vi "Accelerator_DAQ_small.vi"() -> ()   [LabVIEW 2013]
doc: "Acquire Accelerator Data"
uses:
  <instrlib>/niScope/Controls/niScope vertical coupling.ctl
  <instrlib>/niScope/Controls/niScope trigger slope.ctl
  <instrlib>/niScope/Controls/niScope trigger coupling.ctl
  <instrlib>/niScope/Controls/niScope trigger source.ctl
  Accelerator Measurement/Array_Defctl.ctl
  <vilib>/Utility/error.llb/DialogType.ctl
  <vilib>/Utility/miscctls.llb/LVPointTypeDef.ctl
  Public API/Dust_Event.ctl
  Public API/Signal.ctl
  Private/Role ID.ctl
  Private/Hardware ID.ctl
  Private/Estimate_source.ctl
  Functional Global Variables/Action Items.ctl
  <vilib>/Analysis/baseanly.llb/Mean (DBL).vi
  Private/PSU updated.vi
  <vilib>/addons/database/Connection.llb/Conn Execute.vi
  <vilib>/addons/database/Recordset.llb/Rec Fetch Recordset Data (R).vi
  <vilib>/addons/database/Recordset.llb/Rec Destroy - Connection.vi
  <instrlib>/niScope/Configure/Trigger/niScope Configure Trigger Edge.vi
  <instrlib>/niScope/Acquire/Fetch/niScope Multi Fetch Cluster.vi
  <vilib>/addons/database/_DB Variant To Data/Database Variant To Data.xnode
  <vilib>/Analysis/NI_AALBase.lvlib
  <vilib>/addons/database/NI_Database_API.lvlib
panel:
  out "Big Accelerator?":bool
  in  "Trigger":enum32{"Edge"}(tab)
  in  "Trigger Source Edge 2":T1="2" caption="Source"
  in  "Trigger Source Edge":T1="0" caption="Source"
  in  "Coupling":T2=1 items=["AC"=0, "DC"=1, "HF Reject"=3, "LF Reject"=4, "AC Plus HF Reject"=1001]
  in  "Slope":T3 caption="Trigger Slope"
  in  "Level":dbl=1.0 caption="Trigger Level" step=0.001 format="%.3f"
  in  "Delay":dbl caption="Trigger Delay" format="%.4p"
  in  "Reference Position (%)":dbl=40.0 caption="Ref Position" format="%.1f"
  in  "Bandwidth":dbl=-1.0 format="%.2f"
  in  "Vertical Coupling":T4=1 items=["AC", "DC", "Ground"]
  in  "Probe Attenuation":dbl=1.0 format="%.1f"
  in  "Vertical Offset":dbl format="%.4f"
  in  "Vertical Range":dbl=5.0 caption="Vertical Range (V)" format="%.2f"
  out "Actual Sample Rate":dbl=10000000.0 format="%.0p"
  in  "Min Record Length":i32=100000 caption="Min. Record Length"
  in  "Min Sample Rate":dbl=80000000.0 caption="Min. Sample Rate" step=1000000.0 format="%.2p"
  out "Actual Record Length":i32=100000
  out "Mass":dbl format="%#_3g"
  in  "Write to Database?":bool=TRUE
  in  "Limit":dbl
  in  "Limit Triggers":bool
  out "Acquisition #":i32
  in  "WFM Tag":string="trace"
  in  "Location":string="G:\\default"
  in  "Write Raw File?":bool
  out "Saving Raw File...":path=path "G:/2012_06_13_verify_timestamp_labview/trace00000"
  out "?":cluster{dbl, dbl}(knob)={0.0549, 2.0} scale=10.0..0.01
  in  "Ideal Time (Cursor)":dbl=2.0 step=0.01 format="%_2f"
  out "Time Between Triggers":dbl
  out "Average Frequency":dbl format="%#_4g"
  out "output cluster":T5
  out "error out 4":errorcluster
  out "error out 3":errorcluster
  out "# elements in queue":i32
  out "Stop condition":bool=TRUE
  out "created path":path=path "G:/default"
  out "Numeric":i32=92364
  out "error out 2":errorcluster
  out "Calibration":dbl=24700000000000.0
  out "Array":T6=["Dev1", "Dev2"]
  out "Multi Plot 2":cluster{dbl[], dbl[]}(graph) caption="Multi Plot"
  in  "Acceleration Voltage (MV)":dbl=2.0 format="%_2g"
  out "Charge":dbl format="%#_3g"
  out "Velocity (Est.)":dbl format="%#_6f"
  out "Final Detector (CH3)":waveform(dbl)(graph)={"t0"=timestamp(0 s since 1904-01-01), "dt"=1e-07, "Y"=[]}
  out "Charge Detector/PSU gate (CH2)":waveform(dbl)(graph)={"t0"=timestamp(0 s since 1904-01-01), "dt"=1e-07, "Y"=[]}
  out "Velocity Detectors (CH0 & CH1)":waveform(dbl)[](graph)
  in  "stop":bool=TRUE
  out "error out":errorcluster={"status"=FALSE, "code"=0, "source"="No Error"} {"code" format="%.0x"}
  # "File Parameters"
  # "Error Handling"
  # "Trigger"
  # "Channel"
  # "Vertical"
  # "Horizontal"
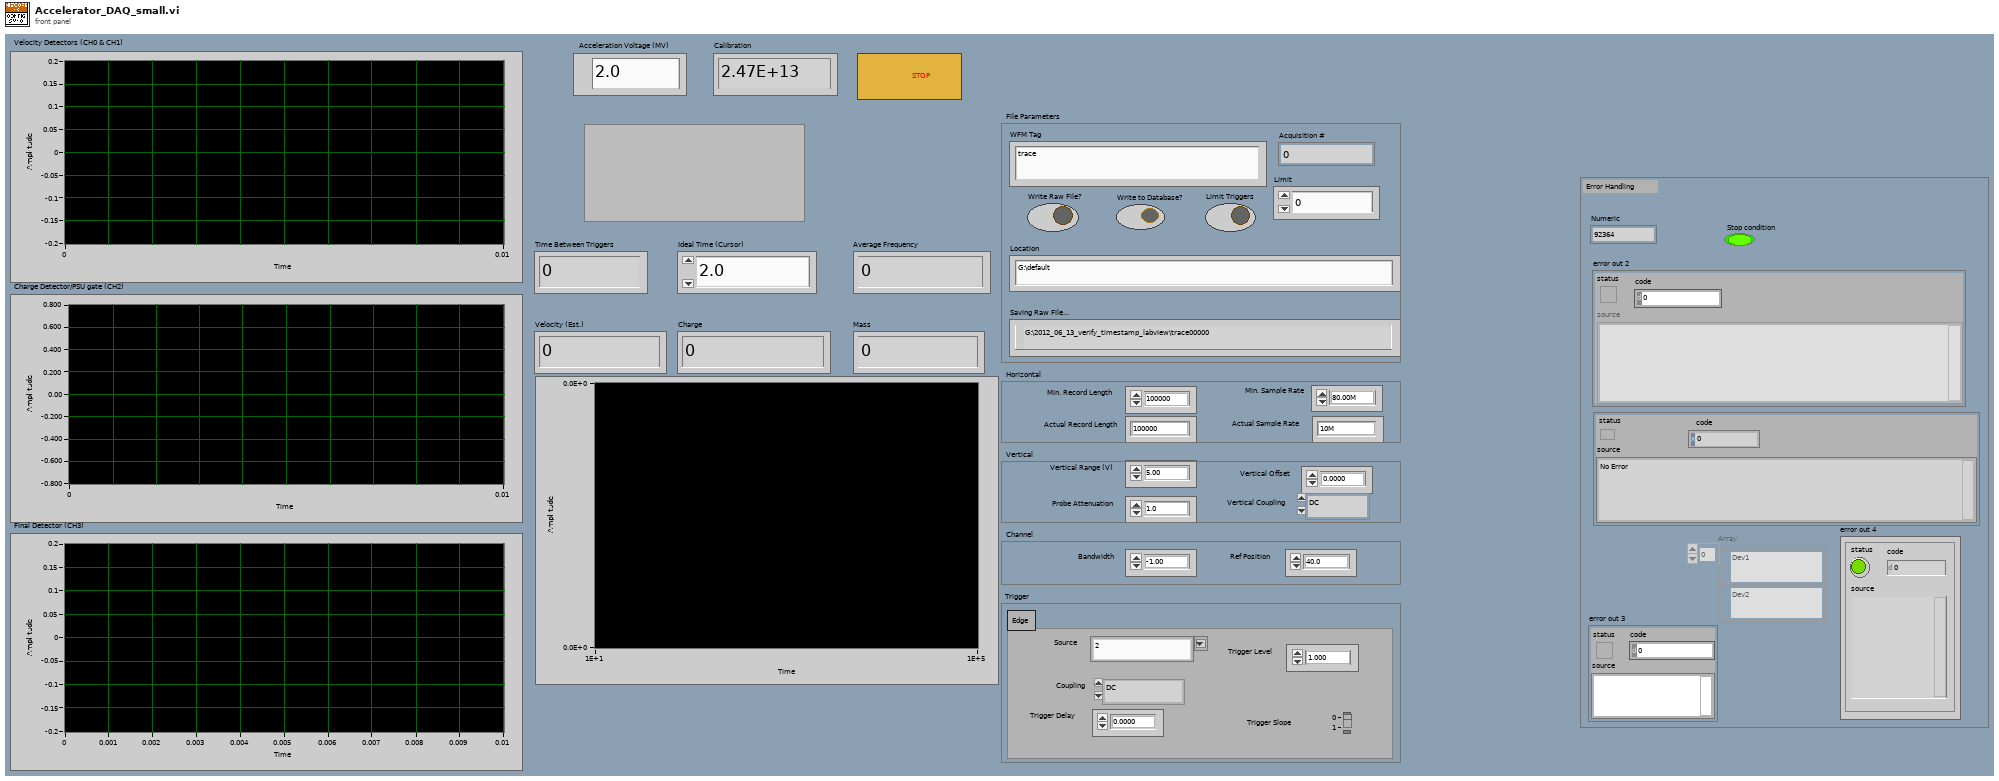
[diagram p1: front panel]
types:
  T1 = typedef "niScope trigger source.ctl" = string
  T2 = typedef "niScope trigger coupling.ctl" = u16
  T3 = typedef "niScope trigger slope.ctl" = i32
  T4 = typedef "niScope vertical coupling.ctl" = i32
  T5 = cluster{"File Path Control":path, "Array":waveform(dbl)[]}
  T6 = typedef "Array_Defctl.ctl" = refnum<k15>[]
  T7 = typedef "LVPointTypeDef.ctl" = cluster{"Horizontal":i16, "Vertical":i16}
  T8 = typedef "DialogType.ctl" = u16
  T9 = typedef "LVAllMonitorsDisplayTypeDef.ctl" = cluster{"Bounds":cluster{"Left":i16, "Top":i16, "Right":i16, "Bottom":i16}, "Depth":i16}[]
  T10 = cluster{"Bounds":cluster{"Left":i16, "Top":i16, "Right":i16, "Bottom":i16}, "Depth":i16}
  T11 = cluster{"Left":i16, "Top":i16, "Right":i16, "Bottom":i16}
  T12 = typedef "NI_Database_API.lvlib/Conn ObjectReference.ctl" = refnum<k1>
  T13 = typedef "NI_Database_API.lvlib/Rec ObjectReference.ctl" = refnum<k1>
  T14 = cluster{"Integer Timestamp":dbl, "Max Velocity":dbl, "Min Velocity":dbl}
  T15 = cluster{"first point time":dbl, "xIncrement":dbl, "Waveforms":dbl[]}[]
  T16 = typedef "Dust_Event.ctl" = cluster{"Time Stamp":timestamp, "Velocity":sgl, "Mass":sgl, "Charge":sgl, "Radius":sgl, "Array":T17[], "Dust Event ID":i64, "Passed_3rd_Detector":bool, "Estimate Source":T20, "Estimate Quality":sgl}
  T17 = typedef "Signal.ctl" = cluster{"Signal ID":i64, "Time Stamp":timestamp, "Dust Event ID":i64, "Role ID":T18, "Data":sgl[], "Signal Length":i32, "dt":sgl, "Offset":dbl, "Hardware ID":T19}
  T18 = typedef "Role ID.ctl" = enum16{"First_Detector", "Second_Detector", "Third_Detector", "LeCroy_CH1", "LeCroy_CH2", "LeCroy_CH3", "LeCroy_CH4", "PSU"}
  T19 = typedef "Hardware ID.ctl" = enum16{"Unknown", "CSA 1", "CSA 2", "CSA 3", "CSA 4", "CSA 5", "CSA 6"}
  T20 = typedef "Estimate_source.ctl" = i8
  T21 = typedef "Action Items.ctl" = enum16{"Initialize", "Get", "Set"}
  T22 = cluster{"relativeInitialX":dbl, "xIncrement":dbl, "wfm":dbl[]}[]
  T23 = cluster{"first point time":dbl, "xIncrement":dbl, "Waveforms":dbl[]}
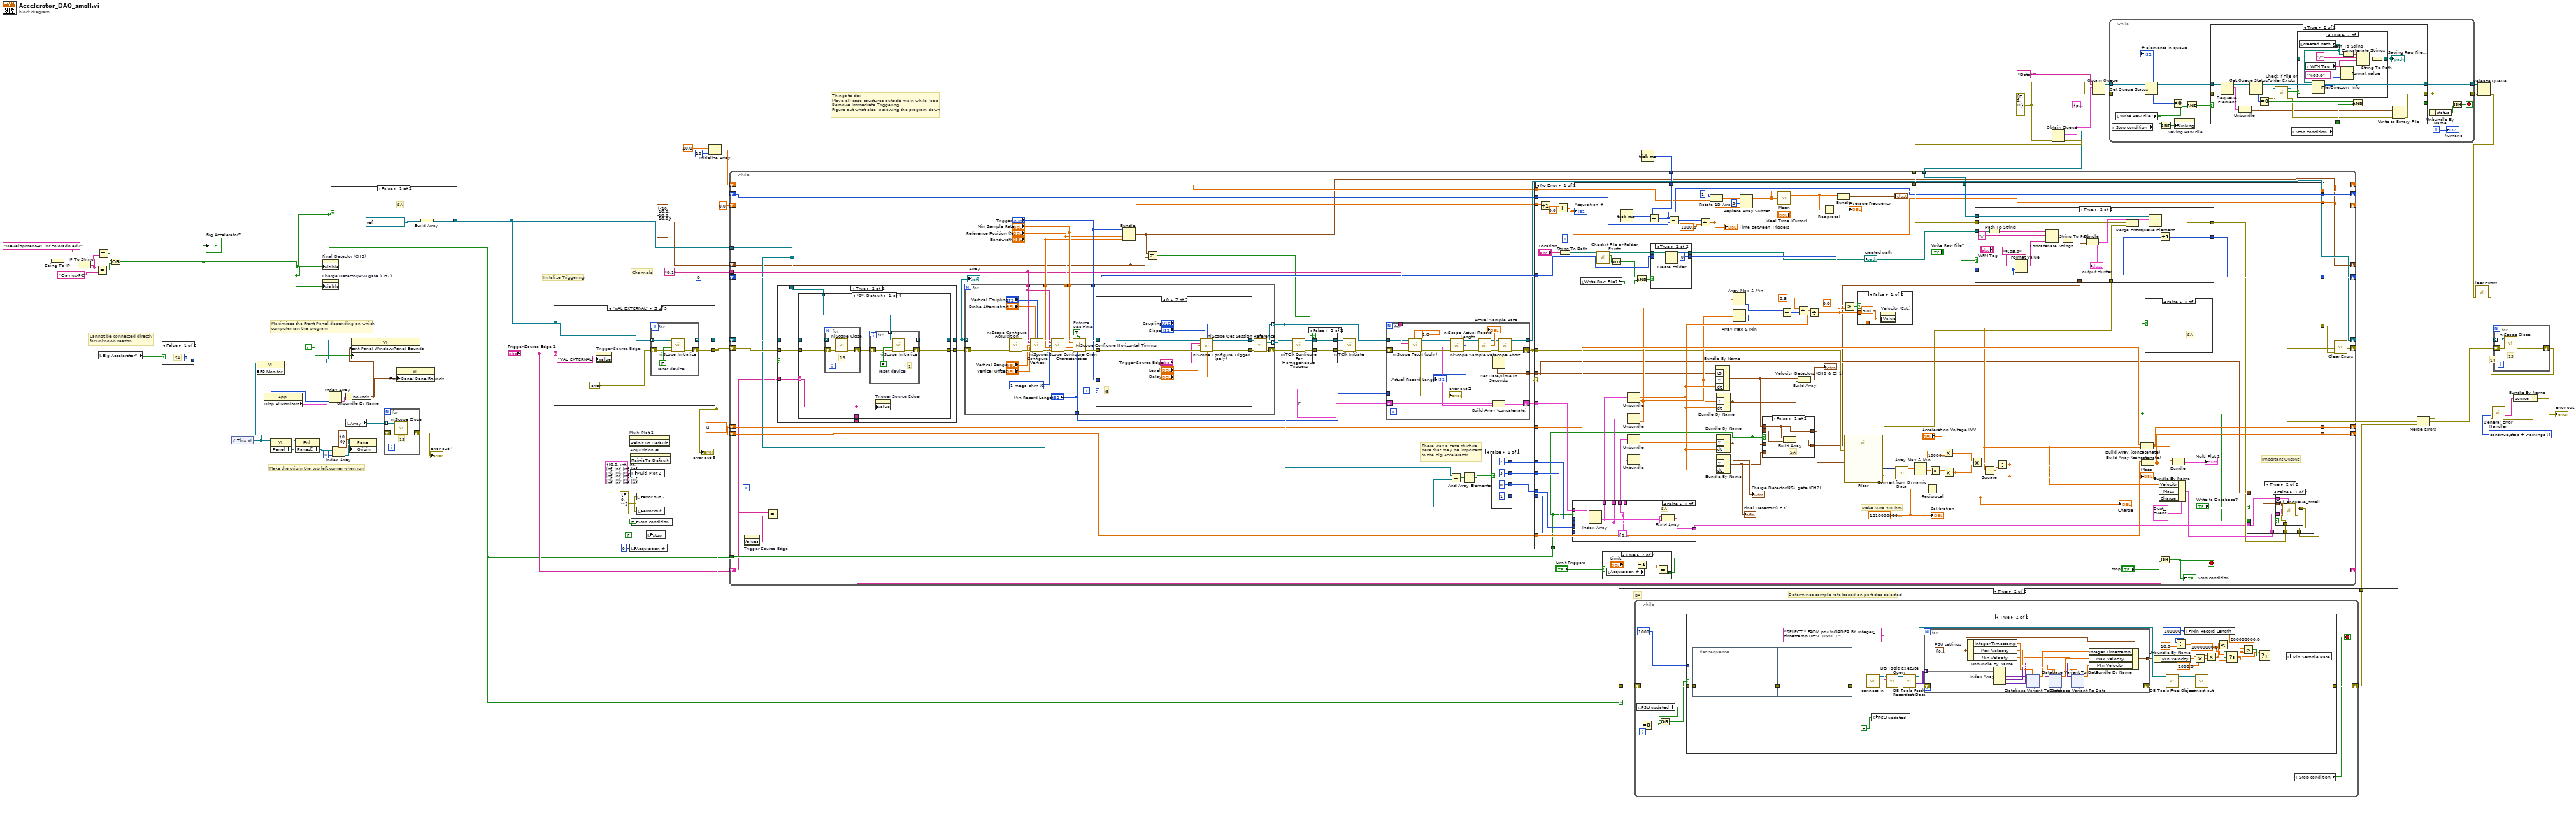
[diagram p0: block diagram]
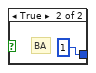
[diagram p2: hidden frame]
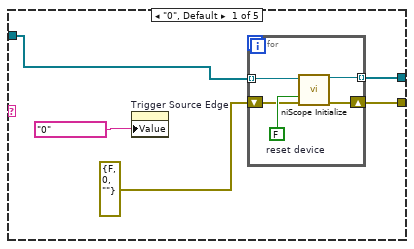
[diagram p3: hidden frame]
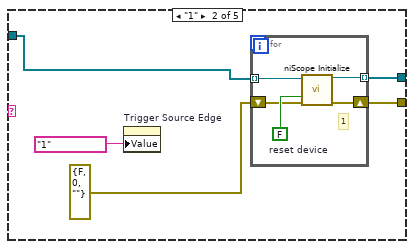
[diagram p4: hidden frame]
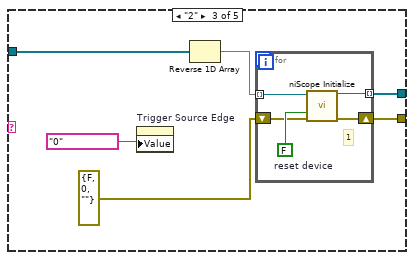
[diagram p5: hidden frame]
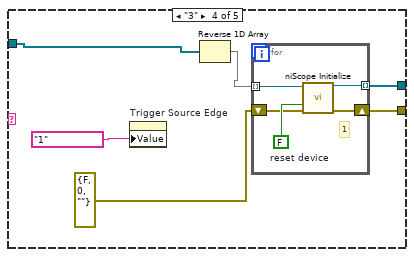
[diagram p6: hidden frame]
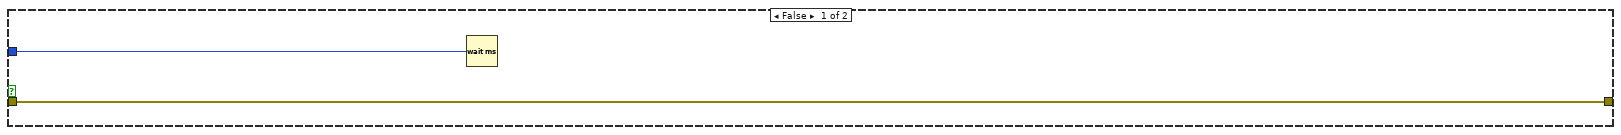
[diagram p8: hidden frame]
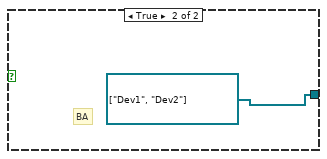
[diagram p9: hidden frame]
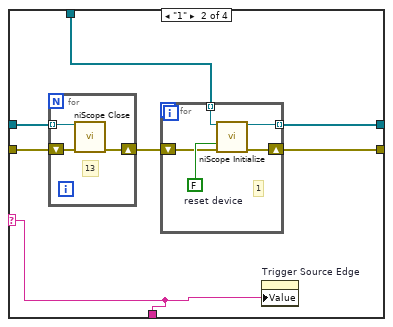
[diagram p11: hidden frame]
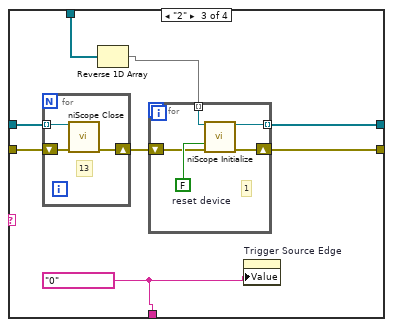
[diagram p12: hidden frame]
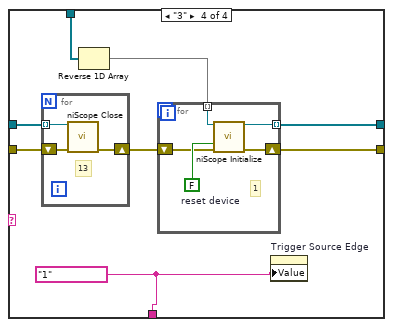
[diagram p13: hidden frame]
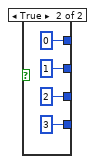
[diagram p14: hidden frame]
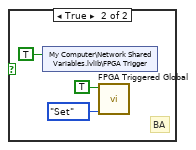
[diagram p16: hidden frame]
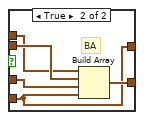
[diagram p17: hidden frame]
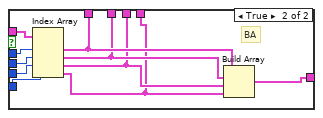
[diagram p18: hidden frame]
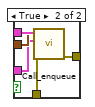
[diagram p20: hidden frame]
diagram:
  w29 = dbl[] []
  w36 = errorcluster {"status"=FALSE, "code"=0, "source"=""} ("error out")
  w41 = errorcluster {"status"=FALSE, "code"=0, "source"=""} ("error out")
  w42 = cluster{path, waveform(sgl)[]} {path "", []} ("output cluster")
  w43 = "Data" ("name (unnamed)")
  w34 = T8 4 items=["no dialog", "OK message", "continue or stop message", "OK message + warnings", "continue/stop + warnings"] ("type of dialog (OK msg:1)")
  # "Cannot be connected directly\nfor unknown reason"
  # "Maximizes the Front Panel depending on which\ncomputer ran the program"
  # "Things to do:\nMove all case structures outside main while loop\nRemove Immediate Triggering\nFigure out what else is slowing the program down"
  # "Channels"
  # "Make the origin the top left corner when run"
  # "Initalize Triggering"
  # "14"
  n1 = String To IP() -> (0:w17:u32)  [unwired: 1 in]
  n2 = IP To String(2:w17) -> (0:w14:string)  [unwired: 1 in]
  n3 = Equal?(x=w14, y="Clavius-PC") -> (x = y?=w4:bool)
  n4 = Equal?(x="Development-PC.int.colorado.edu", y=w14) -> (x = y?=w3:bool)
  n5 = local read "Big Accelerator?"() -> (w1:bool)
  n6 = Or(x=w3, y=w4) -> (x .or. y?=w2:bool)
  "Big Accelerator?" <- w2
  n7 = case shown="False" w1 {
    tunnel: [0 1] -> w10
    frame False {
      # "SA"
    }
    frame True {
      # "BA"
    }
  }
  n8 = control-ref of="This VI"() -> (w11:refnum<vi>)
  n9 = property class="VI"(reference=w11, "FP.Monitor"=w10) -> (reference out=w7:refnum<vi>)  [unwired: 1 in, 1 out]
  n10 = property class="App"() -> ("Disp.AllMonitors"=w9:T9)  [unwired: 2 in, 2 out]
  n11 = property class="VI"(reference=w11) -> (error out=w25:errorcluster, "Panel"=w12:refnum<vi>)  [unwired: 1 in, 1 out]
  n12 = property class="Pnl"(reference=w12, error in=w25) -> (error out=w24:errorcluster, "Panes[]"=w23:refnum<vi>[])  [unwired: 1 out]
  n13 = property on="Final Detector (CH3)" class="WFGraph (strict)"("Visible"=w2) -> ()  [unwired: 2 in, 2 out]
  n14 = property on="Charge Detector/PSU gate (CH2)" class="WFGraph (strict)"("Visible"=w2) -> ()  [unwired: 2 in, 2 out]
  n15 = Index Array(array=w9, index=w10) -> (element=w8:T10)
  n16 = case shown="False" w2 {
    tunnel: [w66 refnum<k15>[] ["Dev1", "Dev2"] ("Resources")] -> w18
    frame False {
      # "SA"
      n17 = Build Array(refnum<k15> "Dev5" ("resource name")) -> (w66:refnum<k15>[])
    }
    frame True {
      # "BA"
    }
  }
  n18 = Index Array(array=w23, index=0) -> (element=w21:refnum<vi>)
  n19 = Unbundle By Name(w8) -> ("Bounds"=w6:T11)
  n20 = local read "Array"() -> (w44:T6)
  n21 = property class="Pane"(reference=w21, error in=w24, "Origin"=T7 {"Horizontal"=0, "Vertical"=0}) -> (error out=w19:errorcluster)  [unwired: 1 out]
  n22 = property class="VI"(reference=w7, "Front Panel Window:Panel Bounds"=w6, "Front Panel Window:Size to Screen (Deprecated)"=TRUE) -> ()  [unwired: 1 in, 2 out]
  n23 = for {
    tunnel: w44 -> [w69] mode=indexing
    shift-right: [w71] -> w39
    shift-left: w19 -> [w70]
    # "13"
    n24 = call <instrlib>:"niScope Close.vi"("instrument handle"=w69, "error in"=w70) -> ("error out"=w71:errorcluster)  [unwired: 13 in]
  }
  "error out 4" <- w39
  n25 = property class="VI"("Front Panel.PanelBounds"=w6) -> ()  [unwired: 2 in, 2 out]
  n26 = case shown="\"VAL_EXTERNAL\"" "Trigger Source Edge 2" {
    tunnel: [w76 w85 w96 w107 w118] -> w62
    tunnel: [w75 w84 w95 w106 w117] -> w27
    tunnel: w18 -> [w72 w82 w92 w103 w114]
    frame "0", Default {
      n27 = property on="Trigger Source Edge" class="CmbBox (strict)"("Value"=T1 "0" ("Trigger Source Edge")) -> ()  [unwired: 2 in, 2 out]
      n28 = for {
        tunnel: w72 -> [w80] mode=indexing
        tunnel: [w78] -> w76 mode=indexing
        shift-right: [w77] -> w75
        shift-left: errorcluster {"status"=FALSE, "code"=0, "source"=""} ("error out") -> [w79]
        w81 = FALSE  # reset device
        n29 = call <instrlib>:"niScope Initialize.vi"("resource name"=w80, "reset device"=w81, "error in"=w79) -> ("instrument handle"=w78:refnum<k15>, "error out"=w77:errorcluster)  [unwired: 11 in]
      }
    }
    frame "1" {
      n30 = property on="Trigger Source Edge" class="CmbBox (strict)"("Value"=T1 "1" ("Trigger Source Edge")) -> ()  [unwired: 2 in, 2 out]
      n31 = for {
        tunnel: w82 -> [w90] mode=indexing
        tunnel: [w88] -> w85 mode=indexing
        shift-right: [w87] -> w84
        shift-left: errorcluster {"status"=FALSE, "code"=0, "source"=""} ("error out") -> [w89]
        w91 = FALSE  # reset device
        # "1"
        n32 = call <instrlib>:"niScope Initialize.vi"("resource name"=w90, "reset device"=w91, "error in"=w89) -> ("instrument handle"=w88:refnum<k15>, "error out"=w87:errorcluster)  [unwired: 11 in]
      }
    }
    frame "2" {
      n33 = property on="Trigger Source Edge" class="CmbBox (strict)"("Value"=T1 "0" ("Trigger Source Edge")) -> ()  [unwired: 2 in, 2 out]
      n34 = Reverse 1D Array(array=w92) -> (reversed array=w93:refnum<k15>[])
      n35 = for {
        tunnel: w93 -> [w101] mode=indexing
        tunnel: [w99] -> w96 mode=indexing
        shift-right: [w98] -> w95
        shift-left: errorcluster {"status"=FALSE, "code"=0, "source"=""} ("error out") -> [w100]
        w102 = FALSE  # reset device
        # "1"
        n36 = call <instrlib>:"niScope Initialize.vi"("resource name"=w101, "reset device"=w102, "error in"=w100) -> ("instrument handle"=w99:refnum<k15>, "error out"=w98:errorcluster)  [unwired: 11 in]
      }
    }
    frame "3" {
      n37 = property on="Trigger Source Edge" class="CmbBox (strict)"("Value"=T1 "1" ("Trigger Source Edge")) -> ()  [unwired: 2 in, 2 out]
      n38 = Reverse 1D Array(array=w103) -> (reversed array=w104:refnum<k15>[])
      n39 = for {
        tunnel: w104 -> [w112] mode=indexing
        tunnel: [w110] -> w107 mode=indexing
        shift-right: [w109] -> w106
        shift-left: errorcluster {"status"=FALSE, "code"=0, "source"=""} ("error out") -> [w111]
        w113 = FALSE  # reset device
        # "1"
        n40 = call <instrlib>:"niScope Initialize.vi"("resource name"=w112, "reset device"=w113, "error in"=w111) -> ("instrument handle"=w110:refnum<k15>, "error out"=w109:errorcluster)  [unwired: 11 in]
      }
    }
    frame "VAL_EXTERNAL" {
      n41 = property on="Trigger Source Edge" class="CmbBox (strict)"("Value"=T1 "VAL_EXTERNAL" ("Trigger Source Edge")) -> ()  [unwired: 2 in, 2 out]
      n42 = for {
        tunnel: w114 -> [w122] mode=indexing
        tunnel: [w120] -> w118 mode=indexing
        shift-right: [w119] -> w117
        shift-left: errorcluster {"status"=FALSE, "code"=0, "source"=""} ("error out") -> [w121]
        w123 = FALSE  # reset device
        n43 = call <instrlib>:"niScope Initialize.vi"("resource name"=w122, "reset device"=w123, "error in"=w121) -> ("instrument handle"=w120:refnum<k15>, "error out"=w119:errorcluster)  [unwired: 11 in]
      }
    }
  }
  "error out 3" <- w27
  n44 = invoke on="Multi Plot 2" class="XYGraph (strict)" method="Reinit To Default"() -> ()  [unwired: 3 in, 3 out]
  n45 = local write "Acquisition #"(0 ("Acquisition #")) -> ()
  n46 = invoke on="Acquisition #" class="DigNum (strict)" method="Reinit To Default"() -> ()  [unwired: 3 in, 3 out]
  n47 = local write "Multi Plot 2"(cluster{dbl[], dbl[]} {[0.0, inf, inf, inf, inf, inf, inf, inf, inf, inf, inf, inf, inf, inf, inf, inf, inf, inf, inf, inf, inf, inf, inf, inf, inf, inf, inf, inf, inf, inf, inf, inf, inf, inf, inf, inf, inf, inf, inf, inf, inf], [0.0, 0.0, 0.0, 0.0, 0.0, 0.0, 0.0, 0.0, 0.0, 0.0, 0.0, 0.0, 0.0, 0.0, 0.0, 0.0, 0.0, 0.0, 0.0, 0.0, 0.0, 0.0, 0.0, 0.0, 0.0, 0.0, 0.0, 0.0, 0.0, 0.0, 0.0, 0.0, 0.0, 0.0, 0.0, 0.0, 0.0, 0.0, 0.0, 0.0, 0.0]} ("Multi Plot 2")) -> ()
  n48 = local write "Stop condition"(FALSE ("x .or. y?")) -> ()
  n49 = local write "error out 2"(w36) -> ()
  n50 = local write "error out"(w36) -> ()
  n51 = local write "stop"(FALSE ("stop")) -> ()
  n52 = Initialize Array(10.0 ("element"), 10 ("dimension size")) -> (w54:dbl[])
  n53 = case shown="True" w2 {
    tunnel: w27 -> [w124 w126]
    tunnel: [w124 w125] -> w26
    frame False {
      # "SA"
    }
    frame True {
      # "BA"
      # "Determines sample rate based on particles selected"
      n54 = while {
        shift-right: [w133] -> w125
        shift-left: w126 -> [w134]
        i -> [w132]
        stop <- w131 stop-if-true
        n55 = global read "PSU updated.vi" "PSU updated"() -> (w130:bool)
        n56 = Equal To 0?(x=w132) -> (x = 0?=w128:bool)
        n57 = Or(x=w130, y=w128) -> (x .or. y?=w129:bool)
        n58 = case shown="True" w129 {
          tunnel: w134 -> [w135 w165]
          tunnel: [w135 w164] -> w133
          tunnel: 1000 -> [w136 _]
          frame False {
            n59 = Wait (ms)(milliseconds to wait=w136) -> ()  [unwired: 1 out]
          }
          frame True {
            w138 = 200000000.0 ("y")
            w141 = 10000000.0 ("y")
            w148 = 100000 ("Min Record Length")
            n60 = flat-sequence {
              tunnel: [w167] -> w166
              tunnel: w165 -> [w167]
              tunnel: w166 -> [w168]
              tunnel: [w168] -> w151
              frame #0 {
              }
              frame #1 {
              }
            }
            n61 = call "connect in.vi"("error in (no error)"=w151) -> ("error out"=w155:errorcluster, "Database Connection"=w154:T12)  [unwired: 6 in, 1 out]
            n62 = global write "PSU updated.vi" "PSU updated"(FALSE ("PSU updated")) -> ()
            n63 = call-poly <vilib>:"DB Tools Execute Query.vi"("error in (no error)"=w155, "SQL query"="SELECT * FROM psu \nORDER BY integer_timestamp DESC LIMIT 1;", "connection reference"=w154) -> ("error out"=w157:errorcluster, "recordset reference"=w156:T13)  [unwired: 5 in]
            n64 = call-poly <vilib>:"DB Tools Fetch Recordset Data.vi"("error in (no error)"=w157, "recordset reference"=w156) -> ("error out"=w163:errorcluster, "recordset data"=w162:variant[][], "recordset reference out"=w158:T13)  [unwired: 3 in]
            n65 = for {
              tunnel: w162 -> [w184] mode=indexing
              shift-right: [w169] -> w152
              shift-left: w163 -> [w180]
              tunnel: [w179] -> w153
              w174 = T14 {"Integer Timestamp"=0.0, "Max Velocity"=0.0, "Min Velocity"=0.0}  # PSU settings
              n66 = Unbundle By Name(w174) -> ("Integer Timestamp"=w178:dbl, "Max Velocity"=w175:dbl, "Min Velocity"=w172:dbl)
              n67 = Index Array(array=w184) -> (element #1=w183:variant, element #2=w182:variant, element #3=w173:variant)  [unwired: 3 in]
              n68 = xnode "Database Variant To Data"("database variant"=w183, "error in"=w180, "type"=w178) -> ("data"=w177:dbl, "error out"=w181:errorcluster)
              n69 = xnode "Database Variant To Data"("database variant"=w182, "error in"=w181, "type"=w175) -> ("data"=w176:dbl, "error out"=w170:errorcluster)
              n70 = xnode "Database Variant To Data"("database variant"=w173, "error in"=w170, "type"=w172) -> ("data"=w171:dbl, "error out"=w169:errorcluster)
              n71 = Bundle By Name(cluster=w174, "Integer Timestamp"=w177, "Max Velocity"=w176, "Min Velocity"=w171) -> (w179:T14)
            }
            n72 = Unbundle By Name(w153) -> ("Min Velocity"=w147:dbl)
            n73 = call-poly <vilib>:"DB Tools Free Object.vi"("error in (no error)"=w152, "recordset reference"=w158) -> ("error out"=w159:errorcluster, "connection reference"=w160:T12)  [unwired: 8 in]
            n74 = Divide(x=w148, y=10.0) -> (x/y=w144:dbl)
            n75 = local write "Min Record Length"(w148) -> ()
            n76 = Multiply(x=w147, y=1000.0) -> (x*y=w145:dbl)
            n77 = call "connect out.vi"("error in (no error)"=w159, "connection reference"=w160) -> ("error out"=w164:errorcluster)  [unwired: 9 in]
            n78 = Multiply(x=w144, y=w145) -> (x*y=w142:dbl)
            n79 = Less?(x=w142, y=w141) -> (x < y?=w143:bool)
            n80 = Select(t=w141, s=w143, f=w142) -> (s? t:f=w140:dbl)
            n81 = Greater?(x=w140, y=w138) -> (0:w139:bool)
            n82 = Select(t=w138, s=w139, f=w140) -> (s? t:f=w137:dbl)
            n83 = local write "Min Sample Rate"(w137) -> ()
          }
        }
        n84 = local read "Stop condition"() -> (w131:bool)
      }
    }
  }
  n85 = Tick Count (ms)() -> (millisecond timer value=w57:u32)
  n86 = Obtain Queue(name (unnamed)=w43, element data type=w42, error in (no error)=w41) -> (queue out=w38:refnum<queue>, error out=w51:errorcluster)  [unwired: 2 in, 1 out]
  n87 = while {
    shift-right: [w299] -> w37
    shift-left: w27 -> [w304]
    shift-right: [w288] -> _
    shift-left: cluster{i32, dbl, dbl, dbl} {-10, -10.0, -10.0, -10.0} -> [w289]
    tunnel: w57 -> [w296]
    shift-right: [w294] -> _
    shift-left: w54 -> [w295]
    shift-right: [w293] -> _
    shift-left: _ -> [w297]
    shift-right: [w327] -> _
    shift-left: w29 -> [w308]
    shift-right: [w326] -> _
    shift-left: w29 -> [w325]
    tunnel: "0,1" ("Channel Name") -> [w324]
    shift-right: [w305] -> w52
    shift-left: w62 -> [w323]
    tunnel: w38 -> [w314]
    tunnel: w51 -> [w313]
    shift-right: [w312] -> _
    shift-left: 0 -> [w311]
    shift-right: [w291] -> _
    shift-left: 0.0 -> [w292]
    tunnel: w18 -> [w290]
    tunnel: w2 -> [w287]
    shift-right: [w282] -> _
    shift-left: "Trigger Source Edge 2" -> [w281]
    stop <- w303 stop-if-true
    # "There was a case stucture\nhere that may be important\nto the Big Accelerator"
    n88 = property on="Trigger Source Edge" class="CmbBox (strict)"() -> ("Value"=w283:T1)  [unwired: 2 in, 2 out]
    n89 = Equal?(x=w281, y=w283) -> (x = y?=w284:bool)
    n90 = case shown="True" w284 {
      tunnel: w323 -> [w342 w349]
      tunnel: [w341 w348] -> w322
      tunnel: [w342 w347] -> w321
      tunnel: w304 -> [w341 w346]
      tunnel: w290 -> [_ w345]
      tunnel: w281 -> [w340 w344]
      tunnel: [w340 w343] -> w282
      frame False {
      }
      frame True {
        n91 = case shown="\"0\", Default" w344 {
          selector: w344 -> [w350 w365 _ _]
          tunnel: w349 -> [w353 w368 w386 w400]
          tunnel: [w355 w370 w384 w401] -> w347
          tunnel: w346 -> [w352 w367 w385 w399]
          tunnel: [w354 w369 w383 w402] -> w348
          tunnel: w345 -> [w351 w366 w381 w398]
          tunnel: [w350 w365 w380 w396] -> w343
          frame "0", Default {
            n92 = for {
              tunnel: w353 -> [w357] mode=indexing
              shift-right: [w359] -> w356
              shift-left: w352 -> [w358]
              # "13"
              n93 = call <instrlib>:"niScope Close.vi"("instrument handle"=w357, "error in"=w358) -> ("error out"=w359:errorcluster)  [unwired: 13 in]
            }
            n94 = for {
              tunnel: [w363] -> w355 mode=indexing
              shift-right: [w362] -> w354
              shift-left: w356 -> [w360]
              tunnel: w351 -> [w361] mode=indexing
              w364 = FALSE  # reset device
              # "1"
              n95 = call <instrlib>:"niScope Initialize.vi"("resource name"=w361, "reset device"=w364, "error in"=w360) -> ("instrument handle"=w363:refnum<k15>, "error out"=w362:errorcluster)  [unwired: 11 in]
            }
            n96 = property on="Trigger Source Edge" class="CmbBox (strict)"("Value"=w350) -> ()  [unwired: 2 in, 2 out]
          }
          frame "1" {
            n97 = for {
              tunnel: w368 -> [w372] mode=indexing
              shift-right: [w374] -> w371
              shift-left: w367 -> [w373]
              # "13"
              n98 = call <instrlib>:"niScope Close.vi"("instrument handle"=w372, "error in"=w373) -> ("error out"=w374:errorcluster)  [unwired: 13 in]
            }
            n99 = for {
              tunnel: [w378] -> w370 mode=indexing
              shift-right: [w377] -> w369
              shift-left: w371 -> [w375]
              tunnel: w366 -> [w376] mode=indexing
              w379 = FALSE  # reset device
              # "1"
              n100 = call <instrlib>:"niScope Initialize.vi"("resource name"=w376, "reset device"=w379, "error in"=w375) -> ("instrument handle"=w378:refnum<k15>, "error out"=w377:errorcluster)  [unwired: 11 in]
            }
            n101 = property on="Trigger Source Edge" class="CmbBox (strict)"("Value"=w365) -> ()  [unwired: 2 in, 2 out]
          }
          frame "2" {
            w380 = T1 "0" ("Trigger Source Edge")
            n102 = for {
              tunnel: w386 -> [w388] mode=indexing
              shift-right: [w390] -> w387
              shift-left: w385 -> [w389]
              # "13"
              n103 = call <instrlib>:"niScope Close.vi"("instrument handle"=w388, "error in"=w389) -> ("error out"=w390:errorcluster)  [unwired: 13 in]
            }
            n104 = Reverse 1D Array(array=w381) -> (reversed array=w382:refnum<k15>[])
            n105 = for {
              tunnel: [w394] -> w384 mode=indexing
              shift-right: [w393] -> w383
              shift-left: w387 -> [w391]
              tunnel: w382 -> [w392] mode=indexing
              w395 = FALSE  # reset device
              # "1"
              n106 = call <instrlib>:"niScope Initialize.vi"("resource name"=w392, "reset device"=w395, "error in"=w391) -> ("instrument handle"=w394:refnum<k15>, "error out"=w393:errorcluster)  [unwired: 11 in]
            }
            n107 = property on="Trigger Source Edge" class="CmbBox (strict)"("Value"=w380) -> ()  [unwired: 2 in, 2 out]
          }
          frame "3" {
            w396 = T1 "1" ("Trigger Source Edge")
            n108 = for {
              tunnel: w400 -> [w404] mode=indexing
              shift-right: [w406] -> w403
              shift-left: w399 -> [w405]
              # "13"
              n109 = call <instrlib>:"niScope Close.vi"("instrument handle"=w404, "error in"=w405) -> ("error out"=w406:errorcluster)  [unwired: 13 in]
            }
            n110 = Reverse 1D Array(array=w398) -> (reversed array=w397:refnum<k15>[])
            n111 = for {
              tunnel: [w410] -> w401 mode=indexing
              shift-right: [w409] -> w402
              shift-left: w403 -> [w407]
              tunnel: w397 -> [w408] mode=indexing
              w411 = FALSE  # reset device
              # "1"
              n112 = call <instrlib>:"niScope Initialize.vi"("resource name"=w408, "reset device"=w411, "error in"=w407) -> ("instrument handle"=w410:refnum<k15>, "error out"=w409:errorcluster)  [unwired: 11 in]
            }
            n113 = property on="Trigger Source Edge" class="CmbBox (strict)"("Value"=w396) -> ()  [unwired: 2 in, 2 out]
          }
        }
      }
    }
    "Array" <- w321
    n114 = for {
      tunnel: w321 -> [w648] mode=indexing
      shift-right: [w626] -> w331
      shift-left: w322 -> [w647]
      tunnel: w324 -> [w639]
      tunnel: "Min Sample Rate" -> [w632]
      tunnel: "Trigger" -> [w631]
      tunnel: "Bandwidth" -> [w629]
      tunnel: "Reference Position (%)" -> [w628]
      tunnel: [w625] -> w316 mode=indexing
      tunnel: [w624] -> w328 mode=indexing
      tunnel: ["Min Record Length"] -> w315
      i -> [w633]
      w621 = u32 0 items=["1 mega ohm"] ("input impedance")
      w646 = TRUE  # Enforce Realtime
      n115 = call <instrlib>:"niScope Configure Acquisition.vi"("instrument handle"=w648, "error in"=w647) -> ("instrument handle out"=w644:refnum<k15>, "error out"=w645:errorcluster)  [unwired: 12 in]
      n116 = call <instrlib>:"niScope Configure Vertical.vi"("instrument handle"=w644, "probe attenuation"="Probe Attenuation", "vertical coupling"="Vertical Coupling", "channels"=w639, "vertical range"="Vertical Range", "vertical offset"="Vertical Offset", "error in"=w645) -> ("instrument handle out"=w643:refnum<k15>, "error out"=w642:errorcluster)  [unwired: 7 in]
      n117 = call <instrlib>:"niScope Configure Chan Characteristics.vi"("instrument handle"=w643, "channels"=w639, "input impedance"=w621, "maximum input frequency"=w629, "error in"=w642) -> ("instrument handle out"=w640:refnum<k15>, "error out"=w641:errorcluster)  [unwired: 9 in]
      n118 = call <instrlib>:"niScope Configure Horizontal Timing.vi"("instrument handle"=w640, "enforce realtime"=w646, "min sample rate"=w632, "reference position"=w628, "error in"=w641, "min record length"="Min Record Length") -> ("instrument handle out"=w635:refnum<k15>, "error out"=w636:errorcluster)  [unwired: 8 in]
      n119 = case shown="0" w633 {
        tunnel: w636 -> [w649 w659]
        tunnel: w635 -> [w650 w658]
        tunnel: [w650 w657] -> w623
        tunnel: [w649 w656] -> w627
        tunnel: w631 -> [_ _]
        frame 1, Default {
        }
        frame 0 {
          # "6"
          n120 = call-poly <instrlib>:"niScope Configure Trigger (poly).vi"("instrument handle"=w658, "trigger slope"="Slope", "trigger coupling"="Coupling", "trigger source"="Trigger Source Edge", "trigger level"="Level", "error in"=w659, "trigger delay"="Delay") -> ("instrument handle out"=w657:refnum<k15>, "error out"=w656:errorcluster)  [unwired: 7 in]
        }
      }
      n121 = call <instrlib>:"niScope Get Session Reference.vi"("instrument handle"=w623, "error in"=w627) -> ("instrument handle out"=w625:refnum<k15>, "session reference"=w624:refnum<k20>, "error out"=w626:errorcluster)  [unwired: 11 in]
    }
    n122 = Bundle(cluster=w289, "Trigger", "Min Sample Rate", "Reference Position (%)", "Bandwidth") -> (w288:cluster{i32, dbl, dbl, dbl})
    n123 = Not Equal?(x=w288, y=w289) -> (x != y?=w306:bool)
    n124 = call <instrlib>:"niTClk Configure For Homogeneous Triggers.vi"("error in (no error)"=w331, "sessions"=w328) -> ("error out"=w330:errorcluster, "sessions out"=w329:refnum<k20>[])  [unwired: 8 in]
    n125 = case shown="False" w306 {
      tunnel: [w618 w620] -> w338
      tunnel: [w617 w619] -> w337
      tunnel: w329 -> [w615 w620]
      tunnel: w330 -> [w616 w619]
      frame True {
        n126 = call <instrlib>:"niTClk Synchronize.vi"("error in (no error)"=w616, "sessions"=w615) -> ("error out"=w617:errorcluster, "sessions out"=w618:refnum<k20>[])  [unwired: 8 in]
      }
      frame False {
      }
    }
    n127 = call <instrlib>:"niTClk Initiate.vi"("error in (no error)"=w337, "sessions"=w338) -> ("error out"=w339:errorcluster)  [unwired: 8 in, 1 out]
    n128 = for {
      tunnel: w324 -> [w610]
      tunnel: w316 -> [w606] mode=indexing
      shift-right: [w614] -> w307
      shift-left: T15 [] ("Waveform Graph") -> [w608]
      shift-right: [w597] -> w300
      shift-left: w339 -> [w607]
      tunnel: w315 -> [_]
      tunnel: [w599] -> w305 mode=indexing
      tunnel: [w605] -> w309
      n129 = call-poly <instrlib>:"niScope Fetch (poly).vi"("timeout"=1.0 ("Timeout (s)"), "error in"=w607, "channels"=w610, "instrument handle"=w606) -> ("error out"=w601:errorcluster, "waveform"=w609:T22, "instrument handle out"=w602:refnum<k15>)  [unwired: 4 in, 1 out]
      "error out 2" <- w601
      n130 = call <instrlib>:"niScope Actual Record Length.vi"("instrument handle"=w602, "error in"=w601) -> ("instrument handle out"=w613:refnum<k15>, "actual record length"=→"Actual Record Length":i32, "error out"=w612:errorcluster)  [unwired: 11 in]
      n131 = call <instrlib>:"niScope Sample Rate.vi"("instrument handle"=w613, "error in"=w612) -> ("instrument handle out"=w600:refnum<k15>, "actual sample rate"=→"Actual Sample Rate":dbl, "error out"=w598:errorcluster)  [unwired: 11 in]
      n132 = Get Date/Time In Seconds() -> (seconds since 1Jan1904=w605:timestamp)
      n133 = Build Array (concatenate)(w608, w609) -> (w614:T22)
      n134 = call <instrlib>:"niScope Abort.vi"("instrument handle"=w600, "error in"=w598) -> ("instrument handle out"=w599:refnum<k15>, "error out"=w597:errorcluster)  [unwired: 12 in]
    }
    n135 = Equal?(x=w316, y=w290) -> (x = y?=w286:bool[])
    n136 = And Array Elements(Boolean array=w286) -> (logical AND=w285:bool)
    n137 = case shown="False" w285 {
      tunnel: [2 ("index") 0 ("index")] -> w320
      tunnel: [3 ("index") 1 ("index")] -> w319
      tunnel: [0 ("index") 2 ("index")] -> w318
      tunnel: [1 ("index") 3 ("index")] -> w317
      frame False {
      }
      frame True {
      }
    }
    n138 = case shown="No Error" w300 {
      tunnel: [w497 w589] -> w327
      tunnel: [w496 w590] -> w326
      tunnel: w325 -> [w495 w590]
      tunnel: w320 -> [w440 _]
      tunnel: w319 -> [w439 _]
      tunnel: w318 -> [w438 _]
      tunnel: w317 -> [w437 _]
      tunnel: w314 -> [w491 _]
      tunnel: w313 -> [w490 _]
      tunnel: [w486 w591] -> w312
      tunnel: w311 -> [w485 w591]
      tunnel: w309 -> [w446 _]
      tunnel: w308 -> [w476 w589]
      tunnel: w307 -> [w441 _]
      tunnel: w300 -> [w467 w588]
      tunnel: [w444 w588] -> w298
      tunnel: w297 -> [w451 w587]
      tunnel: w296 -> [w455 _]
      tunnel: w295 -> [w454 w586]
      tunnel: [w453 w586] -> w294
      tunnel: [w452 w587] -> w293
      tunnel: w292 -> [w448 w585]
      tunnel: [w447 w585] -> w291
      tunnel: w287 -> [w425 _]
      frame No Error {
        w493 = 12100000000000.0 ("x")
        (unwired) 1
        # "Important Output"
        # "Make Sure 50Ohm"
        n139 = Increment(x=w448) -> (x+1=w449:dbl)
        n140 = Add(x=w449, y=0.0) -> (x+y=w447:dbl)
        "Acquisition #" <- w447
        n141 = String To Path(string="Location") -> (path=w488:path)
        n142 = case shown="False" w425 {
          tunnel: w441 -> [w534 w544]
          tunnel: w440 -> [w533 w543]
          tunnel: w439 -> [w532 w542]
          tunnel: w438 -> [_ w541]
          tunnel: w437 -> [_ w540]
          tunnel: [w531 w539] -> w436
          tunnel: [w528 w535] -> w432
          tunnel: [w528 w536] -> w431
          tunnel: [w530 w537] -> w430
          tunnel: [w529 w538] -> w429
          frame False {
            w528 = T23 {"first point time"=0.0, "xIncrement"=0.0, "Waveforms"=[]} ("Waveforms")
            # "SA"
            n143 = Index Array(array=w534, index #1=w533, index #2=w532) -> (element #1=w529:T23, element #2=w530:T23)
            n144 = Build Array(w529, w530) -> (w531:T15)
          }
          frame True {
            # "BA"
            n145 = Index Array(array=w544, index #1=w543, index #2=w542, index #3=w541, index #4=w540) -> (element #1=w538:T23, element #2=w537:T23, element #3=w536:T23, element #4=w535:T23)
            n146 = Build Array(w538, w537, w536, w535) -> (w539:T15)
          }
        }
        n147 = local read "Write Raw File?"() -> (w420:bool)
        n148 = call <vilib>:"Check if File or Folder Exists.vi"("path"=w488) -> ("file or folder exists?"=w424:bool, "dup path"=w421:path)  [unwired: 8 in, 1 out]
        n149 = Not(x=w424) -> (.not. x?=w423:bool)
        n150 = Tick Count (ms)() -> (millisecond timer value=w460:u32)
        n151 = Unbundle(w429) -> ("xIncrement"=w481:dbl, "Waveforms"=w475:dbl[])  [unwired: 1 out]
        n152 = Unbundle(w430) -> ("Waveforms"=w474:dbl[])  [unwired: 2 out]
        n153 = Unbundle(w431) -> ("Waveforms"=w473:dbl[])  [unwired: 2 out]
        n154 = Unbundle(w432) -> ("Waveforms"=w472:dbl[])  [unwired: 2 out]
        n155 = And(x=w423, y=w420) -> (x .and. y?=w422:bool)
        n156 = Subtract(x=w460, y=w455) -> (x-y=w452:u32)
        n157 = case shown="True" w422 {
          tunnel: [w513 w516] -> w477
          tunnel: w421 -> [w513 w515]
          tunnel: w485 -> [w512 _]
          tunnel: [w512 0] -> w484
          frame False {
          }
          frame True {
            n158 = Create Folder(path (use dialog)=w515) -> (created path=w516:path)  [unwired: 2 in, 2 out]
          }
        }
        "created path" <- w477
        n159 = Subtract(x=w452, y=w451) -> (x-y=w461:u32)
        n160 = Divide(x=w461, y=1000.0) -> (x/y=w459:dbl)
        "Time Between Triggers" <- w459
        n161 = Rotate 1D Array(1:w454, 2:1 ("n")) -> (0:w464:dbl[])
        n162 = Bundle By Name("t0"=w446, "Y"=w475, "dt"=w481) -> (w426:waveform(dbl))  [unwired: 1 in]
        n163 = Bundle By Name("Y"=w474, "dt"=w481) -> (w434:waveform(dbl))  [unwired: 1 in]
        n164 = Bundle By Name("Y"=w473, "dt"=w481) -> (w435:waveform(dbl))  [unwired: 1 in]
        "Charge Detector/PSU gate (CH2)" <- w435
        n165 = Bundle By Name("Y"=w472, "dt"=w481) -> (w433:waveform(dbl))  [unwired: 1 in]
        "Final Detector (CH3)" <- w433
        n166 = Array Max & Min(array=w474) -> (min index (indices)=w483:i32)  [unwired: 3 out]
        n167 = Array Max & Min(array=w475) -> (min index (indices)=w482:i32)  [unwired: 3 out]
        n168 = Replace Array Subset(array=w464, new element=w459, index=0) -> (w453:dbl[])
        n169 = case shown="False" w425 {
          tunnel: w435 -> [_ w527]
          tunnel: w434 -> [w521 w526]
          tunnel: w426 -> [w520 w525]
          tunnel: w433 -> [_ w523]
          tunnel: [w522 w524] -> w428
          tunnel: [w520 w523] -> w427
          frame False {
            # "SA"
            n170 = Build Array(w520, w521) -> (w522:waveform(dbl)[])
          }
          frame True {
            # "BA"
            n171 = Build Array(w525, w526, w527, w523) -> (w524:waveform(dbl)[])
          }
        }
        n172 = call-poly <vilib>:"Mean.vi"("X"=w453) -> ("mean"=w458:dbl)  [unwired: 1 out]
        n173 = Subtract(x=w483, y=w482) -> (x-y=w510:i32)
        n174 = Divide(x=0.6, y=w510) -> (x/y=w508:dbl)
        n175 = Build Array(w426, w434) -> (→"Velocity Detectors (CH0 & CH1)":waveform(dbl)[])
        n176 = Divide(x=w508, y=w481) -> (x/y=w506:dbl)
        n177 = Reciprocal(x=w458) -> (1/x=→"Average Frequency":dbl)
        n178 = Bundle("mean"=w458, "Ideal Time (Cursor)"="Ideal Time (Cursor)") -> (→"?":cluster{"mean":dbl, "Ideal Time (Cursor)":dbl})  [unwired: 1 in]
        n179 = Greater?(x=w506, y=0.0 ("x")) -> (0:w507:bool)
        n180 = call "Filter"("error in (no error)"=w467, "Signal"=w427) -> ("error out"=w480:errorcluster, "Filtered Signal"=w494:dynamicdata)  [unwired: 8 in]
        n181 = case shown="False" w507 {
          tunnel: w506 -> [_ w584]
          tunnel: [w583 w584] -> w469
          frame False {
            w583 = 500.0 ("Velocity")
            n182 = property on="Velocity (Est.)" class="DigNum (strict)"("Value"=w583) -> ()  [unwired: 2 in, 2 out]
          }
          frame True {
            "Velocity (Est.)" <- w584
          }
        }
        n183 = call "Convert from Dynamic Data"("Dynamic Data Type"=w494) -> ("Array"=w504:dbl[])  [unwired: 3 in]
        n184 = Array Max & Min(array=w504) -> (min value=w503:dbl)  [unwired: 3 out]
        n185 = Reciprocal(x=w493) -> (1/x=w492:dbl)
        n186 = Absolute Value(x=w503) -> (abs(x)=w502:dbl)
        n187 = Multiply(x="Acceleration Voltage (MV)", y=1000000.0) -> (x*y=w478:dbl)
        n188 = Multiply(x=w502, y=w492) -> (x*y=w470:dbl)
        "Charge" <- w470
        n189 = Multiply(x=w478, y=w470) -> (x*y=w501:dbl)
        n190 = case shown="True" "Write Raw File?" {
          tunnel: w428 -> [_ w566]
          tunnel: [w563 w580] -> w443
          tunnel: w480 -> [w565 w578]
          tunnel: w491 -> [_ w567]
          tunnel: w490 -> [w564 w576]
          tunnel: w477 -> [_ w574]
          tunnel: [w562 w572] -> w486
          tunnel: w484 -> [w562 w571]
          frame False {
            n191 = Merge Errors(w564, w565) -> (w563:errorcluster)
          }
          frame True {
            n192 = Path To String(path=w574) -> (string=w569:string)
            n193 = Format Value(format string="%05.0", value (0)=w571) -> (output string=w573:string)  [unwired: 1 in]
            n194 = Concatenate Strings(w569, "\\" ("string"), "WFM Tag", w573) -> (w582:string)
            n195 = String To Path(string=w582) -> (path=w575:path)
            n196 = Bundle(w575, w566) -> (w577:cluster{path, waveform(dbl)[]})  [unwired: 1 in]
            "output cluster" <- w577
            n197 = Merge Errors(w576, w578) -> (w579:errorcluster)
            n198 = Enqueue Element(queue=w567, element=w577, error in (no error)=w579) -> (error out=w580:errorcluster)  [unwired: 1 in, 2 out]
            n199 = Increment(x=w571) -> (x+1=w572:i32)
          }
        }
        n200 = Square(x=w469) -> (x^2=w500:dbl)
        n201 = Divide(x=w501, y=w500) -> (x/y=w471:dbl)
        "Mass" <- w471
        n202 = Build Array (concatenate)(w476, w469) -> (w497:dbl[])
        n203 = Build Array (concatenate)(w495, w471) -> (w496:dbl[])
        n204 = case shown="False" w425 {
          frame False {
            # "SA"
          }
          frame True {
            # "BA"
            n205 = shared-variable "My Computer\\Network Shared Variables.lvlib\\FPGA Trigger"(TRUE ("FPGA Trigger")) -> ()  [unwired: 1 in, 1 out]
            n206 = call "FPGA Triggered Global.vi"("Action"=Action_Items."Set", "Input"=TRUE) -> ()  [unwired: 9 in, 1 out]
          }
        }
        n207 = Bundle By Name(cluster=T16 {"Time Stamp"=timestamp(0 s since 1904-01-01), "Velocity"=0.0, "Mass"=0.0, "Charge"=0.0, "Radius"=0.0, "Array"=[], "Dust Event ID"=0, "Passed_3rd_Detector"=FALSE, "Estimate Source"=0, "Estimate Quality"=0.0} ("Input Data"), "Velocity"=w469, "Mass"=w471, "Charge"=w470) -> (w445:T16)
        n208 = Bundle "Bundle"(w497, w496) -> (→"Multi Plot 2":cluster{dbl[], dbl[]})  [unwired: 1 in]
        n209 = case shown="True" "Write to Database?" {
          tunnel: w436 -> [_ w551]
          tunnel: w446 -> [_ w550]
          tunnel: w445 -> [_ w549]
          tunnel: [w545 w548] -> w444
          tunnel: w443 -> [w545 w547]
          tunnel: w425 -> [_ w546]
          frame False {
          }
          frame True {
            n210 = case shown="False" w546 {
              tunnel: w551 -> [w552 w561]
              tunnel: w550 -> [w553 w560]
              tunnel: w549 -> [w554 w559]
              tunnel: [w555 w558] -> w548
              tunnel: w547 -> [w556 w557]
              frame False {
                n211 = call "Call_enqueue_small.vi"("Waveform"=w552, "error in"=w556, "Input Data"=w554, "seconds since 1Jan1904"=w553) -> ("error IO"=w555:errorcluster)  [unwired: 7 in]
              }
              frame True {
                n212 = call "Call_enqueue.vi"("Waveform"=w561, "error in"=w557, "Input Data"=w559, "seconds since 1Jan1904"=w560) -> ("error IO"=w558:errorcluster)  [unwired: 7 in]
              }
            }
          }
        }
        "Calibration" <- w493
      }
      frame Error {
      }
    }
    n213 = case shown="True" "Limit Triggers" {
      tunnel: [FALSE w595] -> w302
      frame False {
      }
      frame True {
        n214 = local read "Acquisition #"() -> (w594:i32)
        n215 = Decrement(x="Limit") -> (x-1=w593:dbl)
        n216 = Equal?(x=w593, y=w594) -> (x = y?=w595:bool)
      }
    }
    n217 = Or(x=w302, y="stop") -> (x .or. y?=w303:bool)
    "Stop condition" <- w303
    n218 = call <vilib>:"Clear Errors.vi"("error in (no error)"=w298) -> ("error out"=w299:errorcluster)  [unwired: 6 in]
  }
  n219 = Obtain Queue(name (unnamed)=w43, element data type=w42, error in (no error)=w41) -> (queue out=w49:refnum<queue>, error out=w48:errorcluster)  [unwired: 2 in, 1 out]
  n220 = while {
    tunnel: w49 -> [w667]
    tunnel: w48 -> [w660]
    tunnel: [w676] -> w47
    tunnel: [w674] -> w46
    i -> [w670]
    stop <- w673 stop-if-true
    n221 = local read "Stop condition"() -> (w662:bool)
    n222 = local read "Write Raw File?"() -> (w664:bool)
    n223 = Get Queue Status(queue=w667, error in (no error)=w660) -> (queue out=w661:refnum<queue>, error out=w668:errorcluster, # elements in queue=w666:i32)  [unwired: 1 in, 5 out]
    "# elements in queue" <- w666
    n224 = And(x=w664, y=w662) -> (x .and. y?=w675:bool)
    n225 = Not Equal To 0?(x=w666) -> (x != 0?=w665:bool)
    n226 = property on="Saving Raw File..." class="Path"("Blinking"=w675) -> ()  [unwired: 2 in, 2 out]
    n227 = And(x=w665, y=w664) -> (x .and. y?=w669:bool)
    n228 = local read "Stop condition"() -> (w663:bool)
    n229 = case shown="True" w669 {
      tunnel: w661 -> [w680 w699]
      tunnel: [w678 w697] -> w674
      tunnel: [w679 w695] -> w676
      tunnel: w663 -> [w681 w694]
      tunnel: [w681 w691] -> w671
      tunnel: w668 -> [w677 w687]
      frame False {
        n230 = Flush Queue(queue=w680, error in (no error)=w677) -> (queue out=w679:refnum<queue>, error out=w678:errorcluster)  [unwired: 1 out]
      }
      frame True {
        n231 = Dequeue Element(queue=w699, error in (no error)=w687) -> (queue out=w696:refnum<queue>, element=w698:cluster{path, waveform(sgl)[]}, error out=w685:errorcluster)  [unwired: 1 in, 1 out]
        n232 = Unbundle(w698) -> (w686:path, w682:waveform(sgl)[])
        n233 = Get Queue Status(queue=w696, error in (no error)=w685) -> (queue out=w695:refnum<queue>, error out=w684:errorcluster, # elements in queue=w693:i32)  [unwired: 1 in, 5 out]
        n234 = Equal To 0?(x=w693) -> (x = 0?=w692:bool)
        n235 = call <vilib>:"Check if File or Folder Exists.vi"("error in (no error)"=w684, "path"=w686) -> ("error out"=w683:errorcluster, "file or folder exists?"=w690:bool, "dup path"=w689:path)  [unwired: 7 in]
        n236 = case shown="True" w690 {
          tunnel: w689 -> [w700 _]
          tunnel: [w700 w706] -> w688
          frame False {
          }
          frame True {
            n237 = local read "created path"() -> (w703:path)
            n238 = local read "WFM Tag"() -> (w708:string)
            n239 = File/Directory Info(path=w703) -> (size=w704:i64)  [unwired: 1 in, 6 out]
            n240 = Format Value(format string="%05.0", value (0)=w704) -> (output string=w707:string)  [unwired: 1 in]
            n241 = Path To String(path=w703) -> (string=w701:string)
            n242 = Concatenate Strings(w701, "\\" ("string"), w708, w707) -> (w705:string)
            n243 = String To Path(string=w705) -> (path=w706:path)
          }
        }
        "Saving Raw File..." <- w688
        n244 = And(x=w692, y=w694) -> (x .and. y?=w691:bool)
        n245 = Write to Binary File(file (use dialog)=w688, data=w682, error in=w683) -> (error out=w697:errorcluster)  [unwired: 3 in, 2 out]
      }
    }
    n246 = Unbundle By Name(w674) -> ("status"=w672:bool)
    n247 = Or(x=w671, y=w672) -> (x .or. y?=w673:bool)
    "Numeric" <- w670
  }
  n248 = Release Queue(queue=w47, error in (no error)=w46) -> (error out=w32:errorcluster)  [unwired: 1 in, 2 out]
  n249 = call <vilib>:"Clear Errors.vi"("error in (no error)"=w32) -> ("error out"=w31:errorcluster)  [unwired: 6 in]
  n250 = Merge Errors(w31, w37, w26) -> (w33:errorcluster)
  n251 = for {
    tunnel: w52 -> [w710] mode=indexing
    shift-right: [w712] -> w63
    shift-left: w33 -> [w711]
    # "13"
    n252 = call <instrlib>:"niScope Close.vi"("instrument handle"=w710, "error in"=w711) -> ("error out"=w712:errorcluster)  [unwired: 13 in]
  }
  n253 = call <vilib>:"General Error Handler.vi"("type of dialog (OK msg:1)"=w34, "error in (no error)"=w63) -> ("message"=w59:string, "error out"=w61:errorcluster)  [unwired: 9 in, 3 out]
  n254 = Bundle By Name(cluster=w61, "source"=w59) -> (→"error out":errorcluster)
